vi "Enum.vi"() -> ()   [LabVIEW 2020]
uses:
  Color-Enum.ctl
panel:
  in  "Color Enum":T1
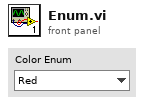
[diagram p1: front panel]
types:
  T1 = typedef "Color-Enum.ctl" = enum16{"Red", "Green", "Blue", "Yellow", "Orange", "Purple"}
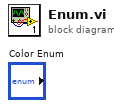
[diagram p0: block diagram]
diagram:
